vi "CSGaussmeter.MaxDisplay.vi"(0 "VisaCluster":T3, 5 "Measurment":string, 7 "Max":T2, 11 "error in (no error)":errorcluster, 12 "Extrem_Max":T1, 13 "Extrem_Min":T1) -> (4 "VisaCluster 2":T3, 6 "Answer":string, 8 "Extrem_Max":T1, 10 "Extrem_Min":T1)   [LabVIEW 2014, in "CSGaussmeter.lvlib"]
uses:
  CSGaussmeter.lvlib
  instr.lib/FH_55/TypeDef/Max.ctl
  instr.lib/FH_55/TypeDef/VisaCluster.ctl
  instr.lib/FH_55/TypeDef/Value_String.ctl
  instr.lib/FH_55/FH 55.lvlib
panel:
  out "Max 2":T2
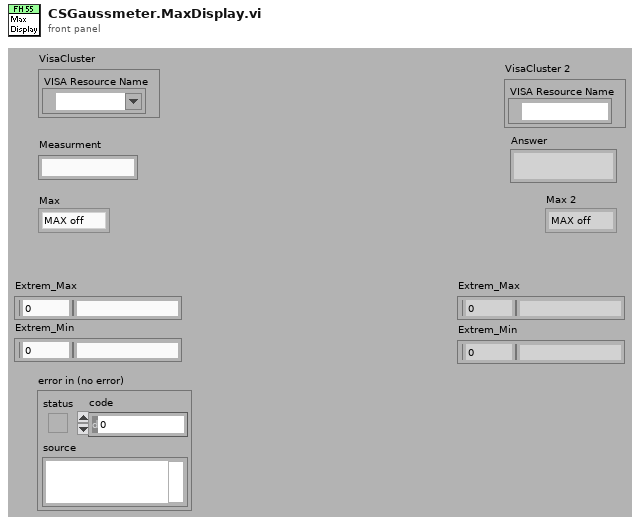
[diagram p1: front panel]
types:
  T1 = typedef "FH 55.lvlib/Value_String.ctl" = cluster{"Numeric":dbl, "String":string}
  T2 = typedef "FH 55.lvlib/Max.ctl" = enum16{"MAX off", "Show MAX", "MAX/MIN"}
  T3 = typedef "FH 55.lvlib/VisaCluster.ctl" = cluster{"VISA Resource Name":refnum<visa-resource-name>}
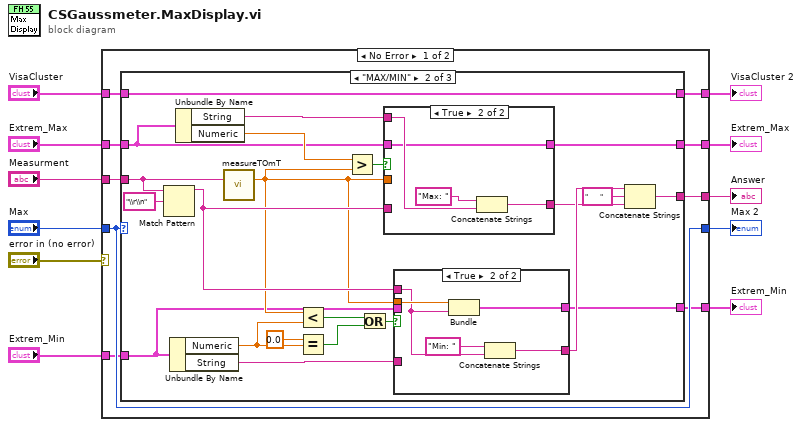
[diagram p0: block diagram]
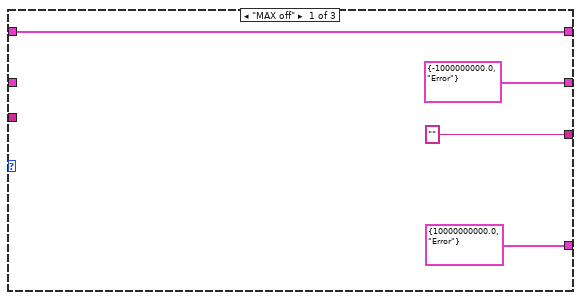
[diagram p2: hidden frame]
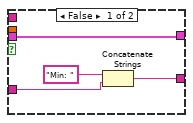
[diagram p3: hidden frame]
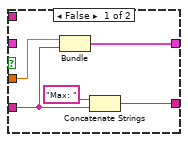
[diagram p4: hidden frame]
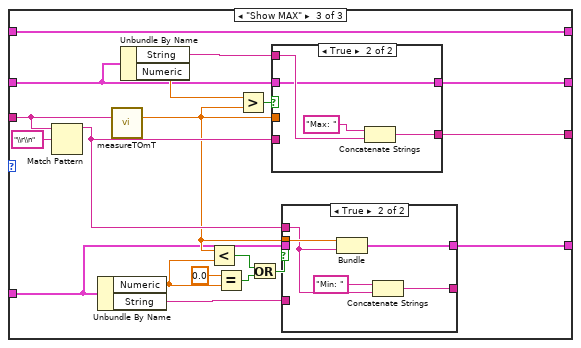
[diagram p5: hidden frame]
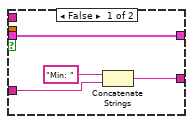
[diagram p6: hidden frame]
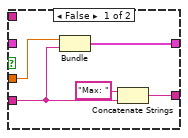
[diagram p7: hidden frame]
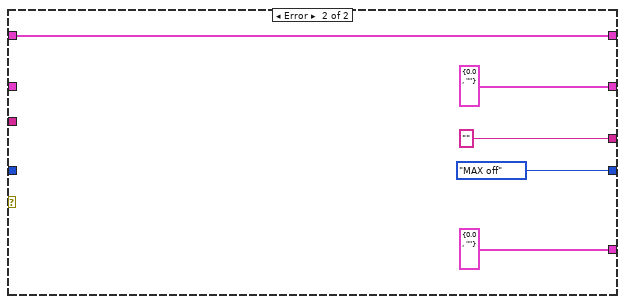
[diagram p8: hidden frame]
diagram:
  n1 = case shown="No Error" "error in (no error)" {
    tunnel: [w17 Max."MAX off" ("Max 2")] -> w11
    tunnel: [w20 "" ("Answer")] -> w10
    tunnel: "VisaCluster" -> [w19 w106]
    tunnel: "Max" -> [w17 _]
    tunnel: [w18 w106] -> w7
    tunnel: "Measurment" -> [w16 _]
    tunnel: "Extrem_Min" -> [w15 _]
    tunnel: "Extrem_Max" -> [w14 _]
    tunnel: [w13 T1 {"Numeric"=0.0, "String"=""} ("Extrem_Max")] -> w2
    tunnel: [w12 T1 {"Numeric"=0.0, "String"=""} ("Extrem_Min")] -> w1
    frame No Error {
      n2 = case shown="\"MAX/MIN\"" w17 {
        tunnel: w19 -> [w23 w43 w80]
        tunnel: ["" w40 w70] -> w20
        tunnel: [w23 w43 w80] -> w18
        tunnel: w16 -> [_ w39 w78]
        tunnel: w15 -> [_ w25 w65]
        tunnel: w14 -> [_ w26 w66]
        tunnel: [T1 {"Numeric"=-1000000000.0, "String"="Error"} ("Extrem_Value") w27 w67] -> w13
        tunnel: [T1 {"Numeric"=10000000000.0, "String"="Error"} ("Extrem_Value") w28 w68] -> w12
        frame "MAX off" {
        }
        frame "MAX/MIN" {
          n3 = Match Pattern(string=w39, regular expression="\\r\\n") -> (before substring=w37:string)  [unwired: 1 in, 3 out]
          n4 = Unbundle By Name(w25) -> ("Numeric"=w35:dbl, "String"=w42:string)
          n5 = Unbundle By Name(w26) -> ("String"=w44:string, "Numeric"=w46:dbl)
          n6 = call "measureTOmT.vi"("string"=w39) -> ("Numeric"=w36:dbl)  [unwired: 12 in, 2 out]
          n7 = Less?(x=w36, y=w35) -> (x < y?=w32:bool)
          n8 = Equal?(x=0.0, y=w35) -> (x = y?=w33:bool)
          n9 = Greater?(x=w46, y=w36) -> (0:w45:bool)
          n10 = Or(x=w32, y=w33) -> (x .or. y?=w31:bool)
          n11 = case shown="True" w45 {
            tunnel: w37 -> [w57 _]
            tunnel: w44 -> [_ w62]
            tunnel: [w60 w63] -> w29
            tunnel: w36 -> [w58 _]
            tunnel: [w56 w61] -> w27
            tunnel: w26 -> [_ w61]
            frame False {
              n12 = Bundle("Numeric"=w58, "Measurment"=w57) -> (w56:cluster{"Numeric":dbl, "Measurment":string})  [unwired: 1 in]
              n13 = Concatenate Strings("Max: " ("string"), w57) -> (w60:string)
            }
            frame True {
              n14 = Concatenate Strings("Max: " ("string"), w62) -> (w63:string)
            }
          }
          n15 = case shown="True" w31 {
            tunnel: w42 -> [w49 _]
            tunnel: [w48 w52] -> w30
            tunnel: w37 -> [_ w53]
            tunnel: w36 -> [_ w54]
            tunnel: [w47 w51] -> w28
            tunnel: w25 -> [w47 _]
            frame False {
              n16 = Concatenate Strings("Min: " ("string"), w49) -> (w48:string)
            }
            frame True {
              n17 = Bundle("Numeric"=w54, "Measurment"=w53) -> (w51:cluster{"Numeric":dbl, "Measurment":string})  [unwired: 1 in]
              n18 = Concatenate Strings("Min: " ("string"), w53) -> (w52:string)
            }
          }
          n19 = Concatenate Strings(w30, "      " ("string"), w29) -> (w40:string)
        }
        frame "Show MAX" {
          n20 = Match Pattern(string=w78, regular expression="\\r\\n") -> (before substring=w76:string)  [unwired: 1 in, 3 out]
          n21 = Unbundle By Name(w65) -> ("Numeric"=w75:dbl, "String"=w79:string)
          n22 = call "measureTOmT.vi"("string"=w78) -> ("Numeric"=w69:dbl)  [unwired: 12 in, 2 out]
          n23 = Unbundle By Name(w66) -> ("String"=w81:string, "Numeric"=w83:dbl)
          n24 = Less?(x=w69, y=w75) -> (x < y?=w72:bool)
          n25 = Equal?(x=0.0, y=w75) -> (x = y?=w73:bool)
          n26 = Greater?(x=w83, y=w69) -> (0:w82:bool)
          n27 = Or(x=w72, y=w73) -> (x .or. y?=w71:bool)
          n28 = case shown="True" w82 {
            tunnel: w76 -> [w94 _]
            tunnel: w81 -> [_ w99]
            tunnel: [w97 w100] -> w70
            tunnel: w69 -> [w95 _]
            tunnel: [w93 w98] -> w67
            tunnel: w66 -> [_ w98]
            frame False {
              n29 = Bundle("Numeric"=w95, "Measurment"=w94) -> (w93:cluster{"Numeric":dbl, "Measurment":string})  [unwired: 1 in]
              n30 = Concatenate Strings("Max: " ("string"), w94) -> (w97:string)
            }
            frame True {
              n31 = Concatenate Strings("Max: " ("string"), w99) -> (w100:string)
            }
          }
          n32 = case shown="True" w71 {
            tunnel: w79 -> [w86 _]
            tunnel: [w85 w89] -> _
            tunnel: w76 -> [_ w90]
            tunnel: w69 -> [_ w91]
            tunnel: [w84 w88] -> w68
            tunnel: w65 -> [w84 _]
            frame False {
              n33 = Concatenate Strings("Min: " ("string"), w86) -> (w85:string)
            }
            frame True {
              n34 = Bundle("Numeric"=w91, "Measurment"=w90) -> (w88:cluster{"Numeric":dbl, "Measurment":string})  [unwired: 1 in]
              n35 = Concatenate Strings("Min: " ("string"), w90) -> (w89:string)
            }
          }
        }
      }
    }
    frame Error {
    }
  }
  "Max 2" <- w11
  "Answer" <- w10
  "VisaCluster 2" <- w7
  "Extrem_Max" <- w2
  "Extrem_Min" <- w1
